vi "Apply gains.vi"(6 "Initalise":bool, 7 "Zero?":bool, 8 "error in (no error)":errorcluster, 11 "Voltage":dbl) -> (0 "error out":errorcluster, 3 "Numeric":dbl)   [LabVIEW 2016]
uses:
  Controls/Gain modes.ctl
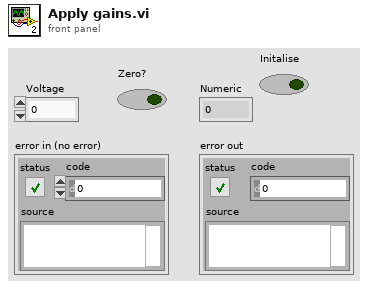
[diagram p1: front panel]
types:
  T1 = typedef "Gain modes.ctl" = enum16{"Initalise", "Get", "Set"}
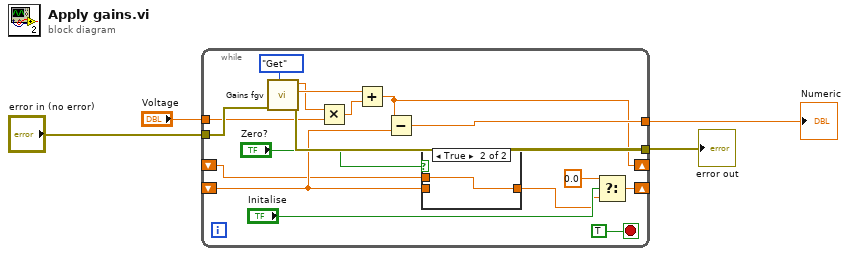
[diagram p0: block diagram]
diagram:
  n1 = while {
    tunnel: "error in (no error)" -> [w20]
    tunnel: [w21] -> w3
    tunnel: "Voltage" -> [w17]
    tunnel: [w7] -> w4
    shift-right: [w10] -> _
    shift-left: _ -> [w12]
    shift-right: [w5] -> _
    shift-left: _ -> [w6]
    stop <- TRUE stop-if-true
    n2 = call "Gains fgv.vi"("Mode"=Gain_modes."Get", "error in (no error)"=w20) -> ("error out"=w21:errorcluster, "Offset"=w19:dbl, "Gain"=w16:dbl)  [unwired: 7 in]
    n3 = Multiply(x=w16, y=w17) -> (x*y=w18:dbl)
    n4 = Add(x=w19, y=w18) -> (x+y=w5:dbl)
    n5 = Subtract(x=w5, y=w12) -> (x-y=w7:dbl)
    n6 = case shown="True" "Zero?" {
      tunnel: w6 -> [_ w23]
      tunnel: w12 -> [w22 _]
      tunnel: [w22 w23] -> w11
      frame False {
      }
      frame True {
      }
    }
    n7 = Select(t=0.0, s="Initalise", f=w11) -> (s? t:f=w10:dbl)
  }
  "Numeric" <- w4
  "error out" <- w3
